vi "Average Waveforms.vi"(8 "error in":errorcluster, 9 "Result Live Graph Plotter in":refnum<class "Live Graph Plotter.lvclass">, 10 "Waveforms Selection":T1={"Record Start Index (0)"=0, "Record Length (-1)"=-1, "Channel List (All)"=""}, 11 "Original Live Graph Plotter in":refnum<class "Live Graph Plotter.lvclass">) -> (0 "error out":errorcluster, 1 "Result Live Graph Plotter out":refnum<class "Live Graph Plotter.lvclass">)   [LabVIEW 2025]
uses:
  Live Graph Plotter/Live Graph Plotter.lvclass
  <vilib>/Analysis/NI_AALBase.lvlib
  <vilib>/Analysis/baseanly.llb/Mean (DBL).vi
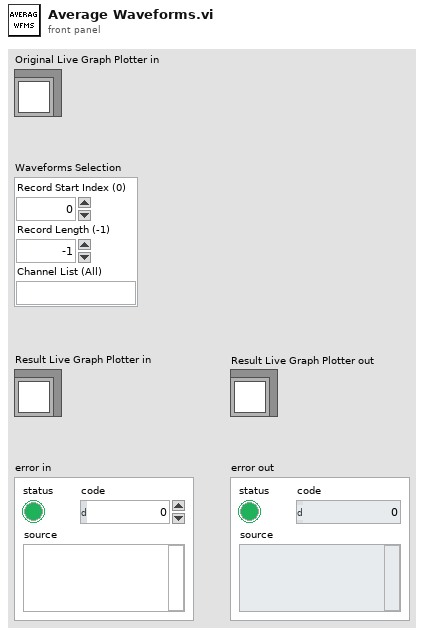
[diagram p1: front panel]
types:
  T1 = cluster{"Record Start Index (0)":i32, "Record Length (-1)":i32, "Channel List (All)":string}
  T2 = cluster{"Channel Name":string, "relativeInitialX":dbl, "xIncrement":dbl, "Waveforms":cluster{"wfm":dbl[]}[]}[]
  T3 = cluster{"relativeInitialX":dbl, "xIncrement":dbl, dbl[]}
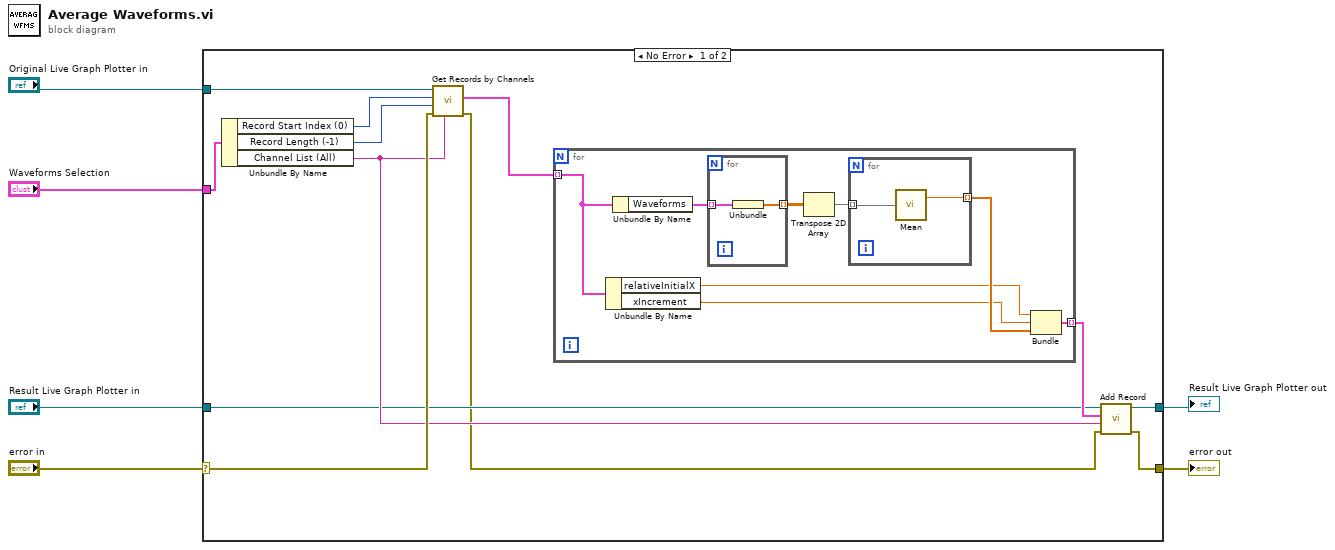
[diagram p0: block diagram]
diagram:
  n1 = case shown="No Error" "error in" {
    selector: "error in" -> [w17 w31]
    tunnel: "Original Live Graph Plotter in" -> [w18 _]
    tunnel: [w7 w31] -> w4
    tunnel: "Waveforms Selection" -> [w16 _]
    tunnel: "Result Live Graph Plotter in" -> [w10 w32]
    tunnel: [w9 w32] -> w1
    frame No Error {
      n2 = Unbundle By Name(w16) -> ("Record Start Index (0)"=w15:i32, "Record Length (-1)"=w12:i32, "Channel List (All)"=w11:string)
      n3 = call "Get Records by Channels.vi"("Channel List (All)"=w11, "error in (no error)"=w17, "Record Length (-1)"=w12, "Record Start Index (0)"=w15, "Live Graph Plotter in"=w18) -> ("error out"=w8:errorcluster, "Records By Channels"=w14:T2)  [unwired: 4 in, 1 out]
      n4 = for {
        tunnel: w14 -> [w22] mode=indexing
        tunnel: [w19] -> w13 mode=indexing
        n5 = Unbundle By Name(w22) -> ("relativeInitialX"=w21:dbl, "xIncrement"=w20:dbl)
        n6 = Unbundle By Name(w22) -> ("Waveforms"=w26:cluster{"wfm":dbl[]}[])
        n7 = for {
          tunnel: w26 -> [w30] mode=indexing
          tunnel: [w29] -> w25 mode=indexing
          n8 = Unbundle(w30) -> ("wfm"=w29:dbl[])
        }
        n9 = Transpose 2D Array(2D array=w25) -> (transposed array=w24:dbl[][])
        n10 = for {
          tunnel: w24 -> [w28] mode=indexing
          tunnel: [w27] -> w23 mode=indexing
          n11 = call-poly <vilib>:"Mean.vi"("X"=w28) -> ("mean"=w27:dbl)  [unwired: 1 out]
        }
        n12 = Bundle("relativeInitialX"=w21, "xIncrement"=w20, w23) -> (w19:T3)  [unwired: 1 in]
      }
      n13 = call "Add Record.vi"("error in (no error)"=w8, "Channel List"=w11, "Waveforms"=w13, "Live Graph Plotter in"=w10) -> ("error out"=w7:errorcluster, "Live Graph Plotter out"=w9:refnum<class "Live Graph Plotter.lvclass">)  [unwired: 6 in]
    }
    frame Error {
    }
  }
  "error out" <- w4
  "Result Live Graph Plotter out" <- w1
